vi "Get Broadcast Events Recursively.vi"(8 "error in (no error)":errorcluster, 11 "Application in":refnum<class "Application.lvclass">) -> (0 "error out":errorcluster, 2 "Broadcast Event":refnum<user-event>[](array[refnum]), 3 "Application out":refnum<class "Application.lvclass">)   [LabVIEW 2020, in "Application.lvclass"]
doc: "Recursively get the broadcast event used to send broadcasts to registered observers."
uses:
  Application.lvclass
  C:/Users/anton/Documents/GitHub/Triarc-Framework/source/Framework/Process/Process.lvclass
  Process/Protected/Broadcasting/Broadcast Message Cluster.ctl
  Process/Process.lvclass/Process.ctl
  Application.lvclass/Application.ctl
  Process/Public/Lifecycle/Get Lifecycle State.vi
  Process/Protected/Messaging/Request Message.vi
  Private/Add Process to Map.vi
  <vilib>/Utility/error.llb/Clear Errors.vi
  Process/Private/SubVIs/Enqueue Request Message.vi
  <vilib>/Utility/error.llb/Error Cluster From Error Code.vi
  Process/Private/SubVIs/Wait for Response Message.vi
  Process/Process.lvclass
  C:/Users/anton/Documents/GitHub/Triarc-Framework/source/Framework/Base/Base.lvclass
  C:/Users/anton/Documents/GitHub/Triarc-Framework/source/Framework/Error Handler Interface/Error Handler Interface.lvclass
  C:/Users/anton/Documents/GitHub/Triarc-Framework/source/Framework/Logging/Logging.lvclass
  C:/Users/anton/Documents/GitHub/Triarc-Framework/source/Framework/Application/Application.lvclass
  C:/Users/anton/Documents/GitHub/Triarc-Framework/source/Framework/Asynchronous Action/Async Action.lvclass
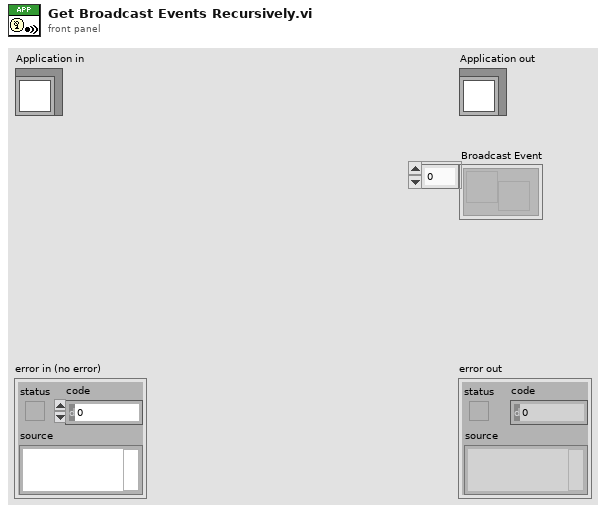
[diagram p1: front panel]
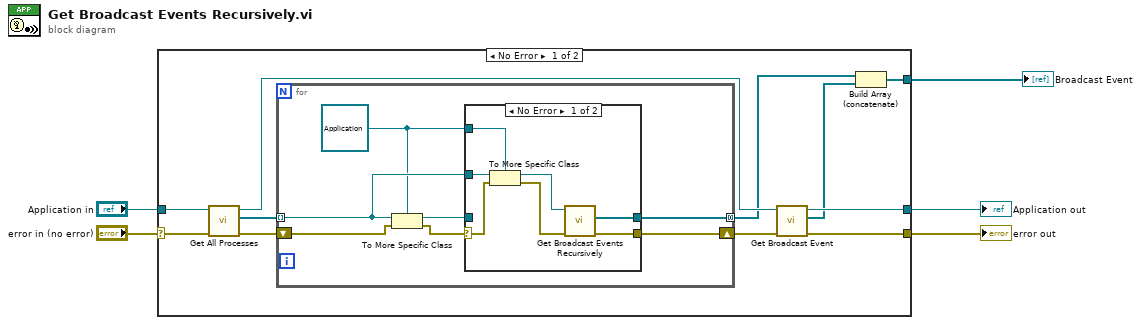
[diagram p0: block diagram]
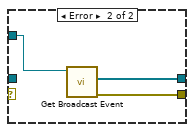
[diagram p2: hidden frame]
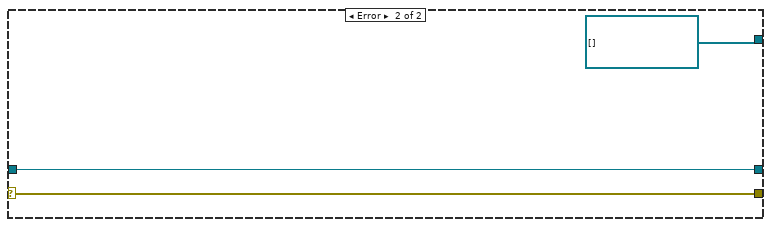
[diagram p3: hidden frame]
diagram:
  n1 = case shown="No Error" "error in (no error)" {
    selector: "error in (no error)" -> [w6 w34]
    tunnel: [w16 w36] -> w5
    tunnel: [w15 refnum<user-event>[] []] -> w4
    tunnel: [w14 w34] -> w3
    tunnel: "Application in" -> [w7 w36]
    frame No Error {
      n2 = call "Get All Processes.vi"("error in (no error)"=w6, "Application In"=w7) -> ("error out"=w8:errorcluster, "App Processes"=w13:refnum<class "Process.lvclass">[], "Application Out"=w12:refnum<class "Application.lvclass">)  [unwired: 7 in]
      n3 = for {
        tunnel: w13 -> [w18] mode=indexing
        tunnel: [w22] -> w11 mode=concatenating
        shift-right: [w23] -> w9
        shift-left: w8 -> [w20]
        w17 = refnum<class "Application.lvclass"> refnum ("Application Out")
        n4 = To More Specific Class(target class=w17, reference=w18, error in=w20) -> (specific class reference=w21:refnum<class "Application.lvclass">, error out=w19:errorcluster)
        n5 = case shown="No Error" w19 {
          selector: w19 -> [w25 _]
          tunnel: [w30 w31] -> w23
          tunnel: [w29 w32] -> w22
          tunnel: w21 -> [_ _]
          tunnel: w18 -> [w28 w33]
          tunnel: w17 -> [w27 _]
          frame No Error {
            n6 = To More Specific Class(target class=w27, reference=w28, error in=w25) -> (specific class reference=w26:refnum<class "Application.lvclass">, error out=w24:errorcluster)
            n7 = call "Get Broadcast Events Recursively.vi"("error in (no error)"=w24, "Application in"=w26) -> ("error out"=w30:errorcluster, "Broadcast Event"=w29:refnum<user-event>[])  [unwired: 7 in, 1 out]
          }
          frame Error {
            n8 = call "Get Broadcast Event.vi"("Process in"=w33) -> ("error out"=w31:errorcluster, "Broadcast Event"=w32:refnum<user-event>[])  [unwired: 8 in, 1 out]
          }
        }
      }
      n9 = call "Get Broadcast Event.vi"("error in (no error)"=w9, "Process in"=w12) -> ("error out"=w14:errorcluster, "Broadcast Event"=w10:refnum<user-event>[], "Process out"=w16:refnum<class "Application.lvclass">)  [unwired: 7 in]
      n10 = Build Array (concatenate)(w11, w10) -> (w15:refnum<user-event>[])
    }
    frame Error {
    }
  }
  "error out" <- w3
  "Application out" <- w5
  "Broadcast Event" <- w4
